vi "Sonicator Settings Dialog.vi"(8 "error in (no error)":errorcluster, 11 "Scale Module Config In":T1={"GUID"="", "Drop Coords"={"Horizontal"=0, "Vertical"=0}, "Process Name"="", "Queue Name"="", "Settings"={"Cycle Period"=500.0, "Mettler"={"VISA resource name"="", "Simulated?"=FALSE}, "Scale Type"=""}, "Load Count"=0}) -> (0 "error out":errorcluster, 1 "Cancelled?":bool=TRUE, 2 "UI Refresh Needed?":bool, 3 "Scale Module Config Out":T1={"GUID"="", "Drop Coords"={"Horizontal"=0, "Vertical"=0}, "Process Name"="", "Queue Name"="", "Settings"={"Cycle Period"=500.0, "Mettler"={"VISA resource name"="", "Simulated?"=FALSE}, "Scale Type"=""}, "Load Count"=0})   [LabVIEW 2018, in "Sonicator Module.lvlib"]
doc: "Dialog for selecting user specified settings."
uses:
  Sonicator Module.lvlib
  Feed Module/Controls/Sonicator Module Settings Cluster.ctl
  Mettler Toledo/Controls/Settings Cluster.ctl
  Feed Module/Controls/Sonicator Module Config Cluster.ctl
  <vilib>/Utility/miscctls.llb/LVPoint32TypeDef.ctl
  <vilib>/Utility/xml.llb/Write to XML File(string).vi
  Settings/Settings.lvlib
  Mettler Toledo/Mettler Toledo.lvlib
panel:
  in  "Module Name":string
  in  "Scale Configurations":T3={"Cycle Period"=500.0, "Mettler"={"VISA resource name"="", "Simulated?"=FALSE}, "Scale Type"="Default"}
  in  "Cancel Button":bool
  in  "OK Button":bool
  # "Non visible portion of dialog (needed for connector pane)."
  # "Scale Settings"
  # "Scale Settings"
  # "Scale Settings"
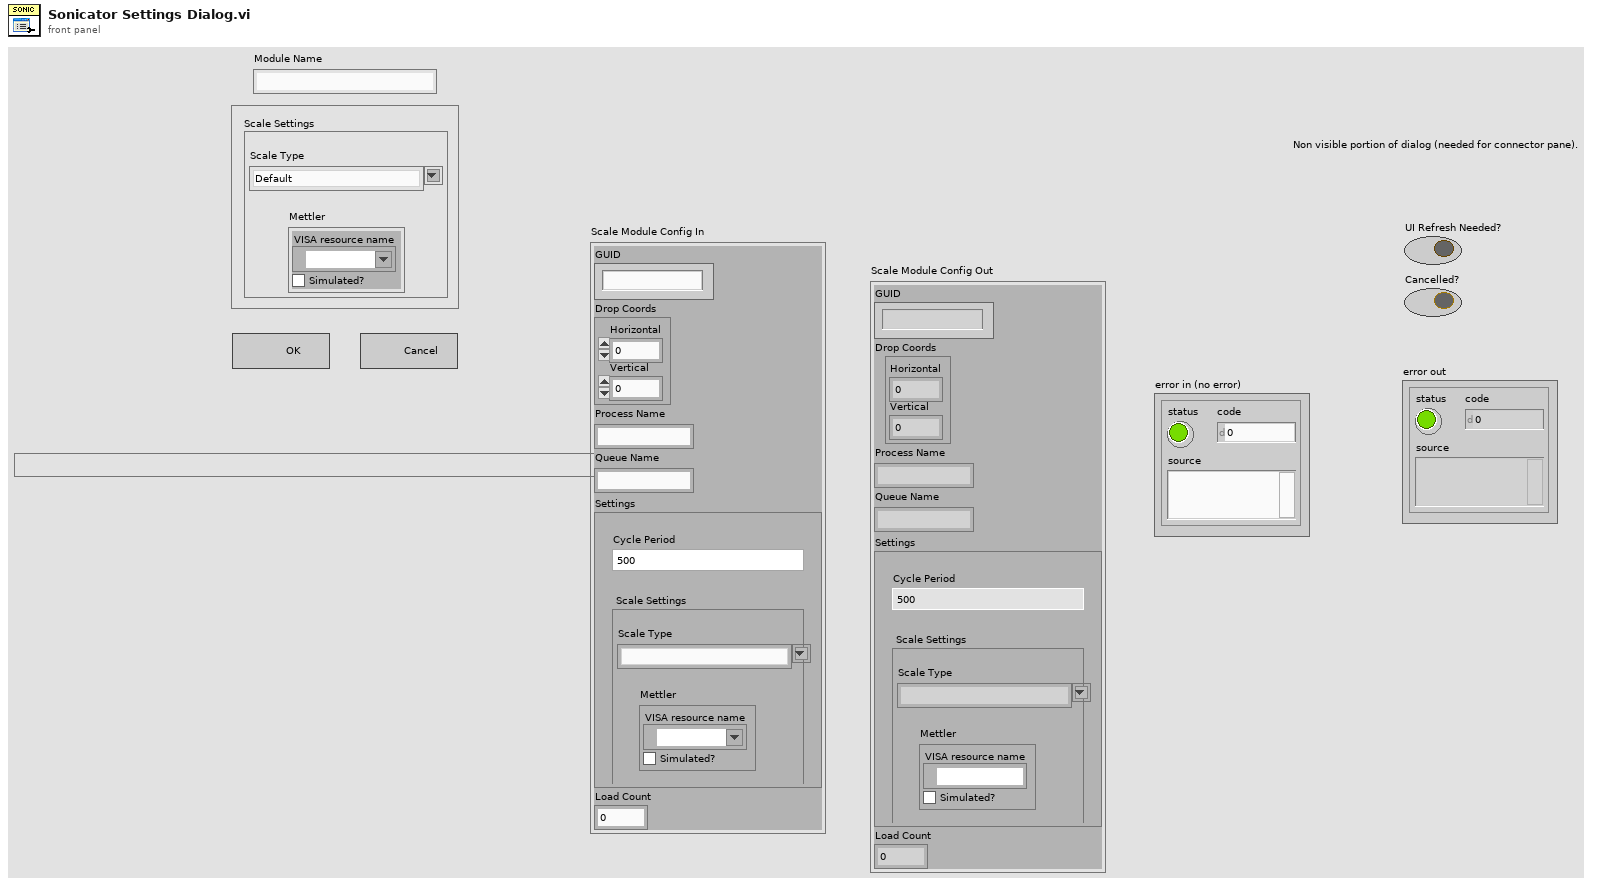
[diagram p1: front panel]
types:
  T1 = typedef "Sonicator Module.lvlib/Sonicator Module Config Cluster.ctl" = cluster{"GUID":string, "Drop Coords":T2, "Process Name":string, "Queue Name":string, "Settings":T3, "Load Count":i32}
  T2 = typedef "LVPoint32TypeDef.ctl" = cluster{"Horizontal":i32, "Vertical":i32}
  T3 = typedef "Sonicator Module.lvlib/Sonicator Module Settings Cluster.ctl" = cluster{"Cycle Period":dbl, "Mettler":T4, "Scale Type":string}
  T4 = typedef "Mettler Toledo.lvlib/Settings Cluster.ctl" = cluster{"VISA resource name":refnum<visa-resource-name>, "Simulated?":bool}
  T5 = enum8{"Enabled", "Disabled", "Disabled and Grayed Out"}
  T6 = cluster{"Cycle Period":dbl, "Mettler":T4, "Scale Type":string}
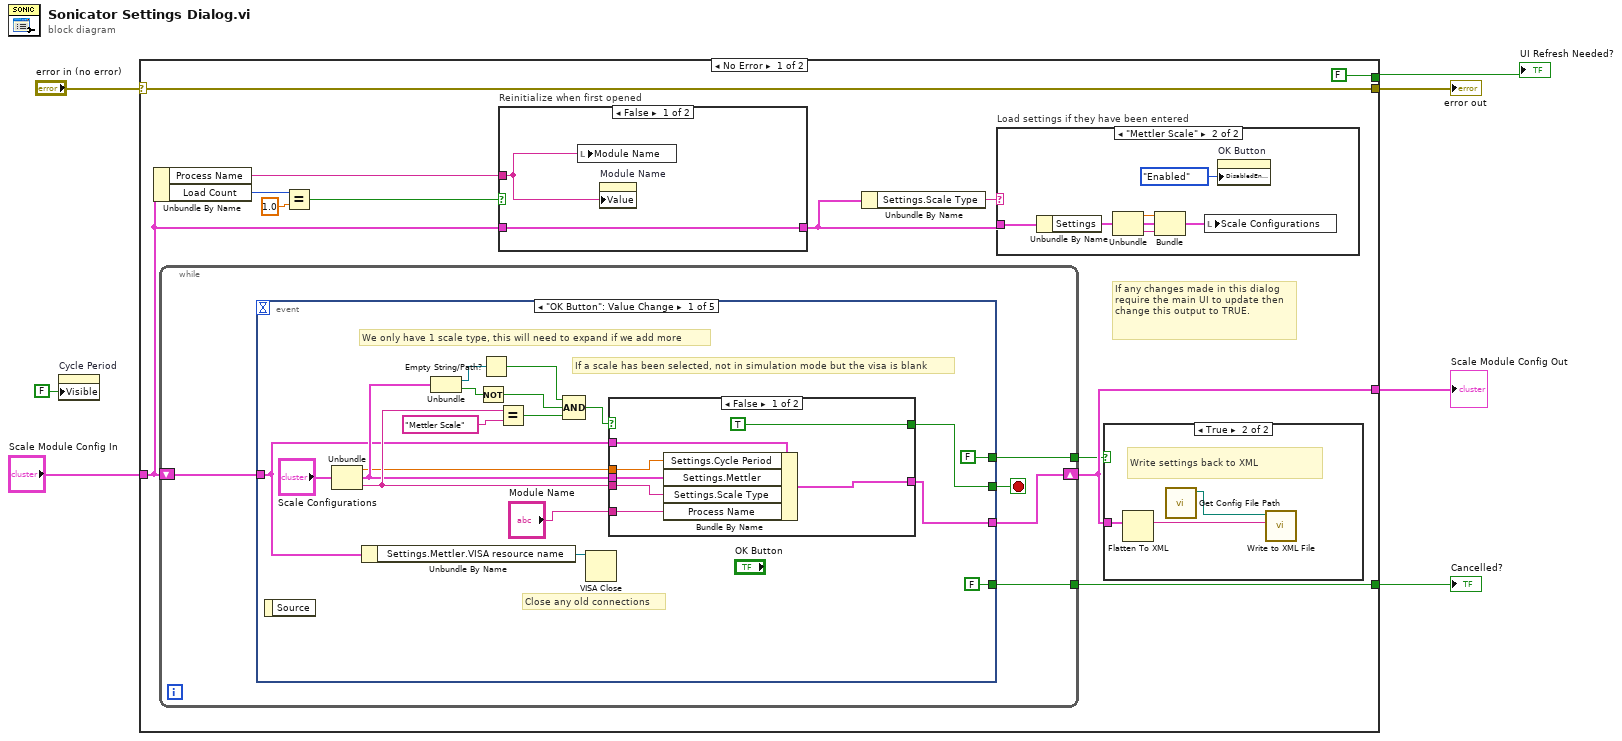
[diagram p0: block diagram]
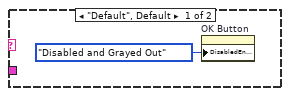
[diagram p2: hidden frame]
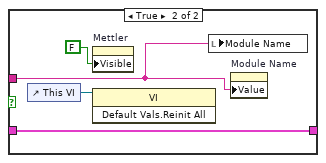
[diagram p3: hidden frame]
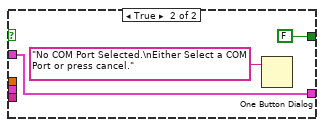
[diagram p4: hidden frame]
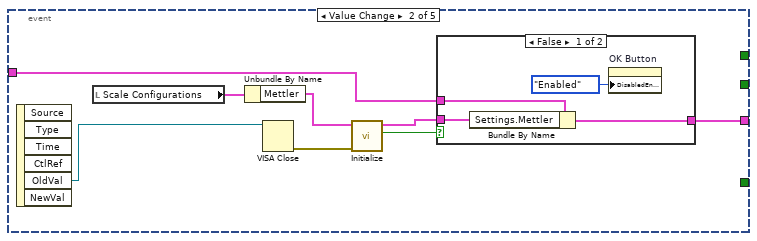
[diagram p5: hidden frame]
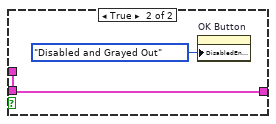
[diagram p6: hidden frame]
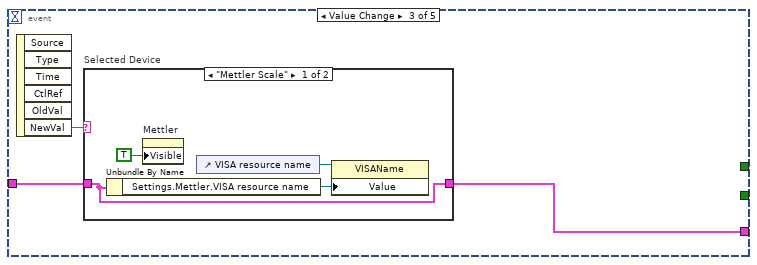
[diagram p7: hidden frame]
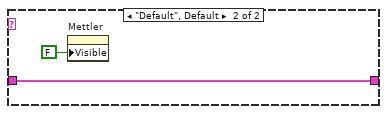
[diagram p8: hidden frame]
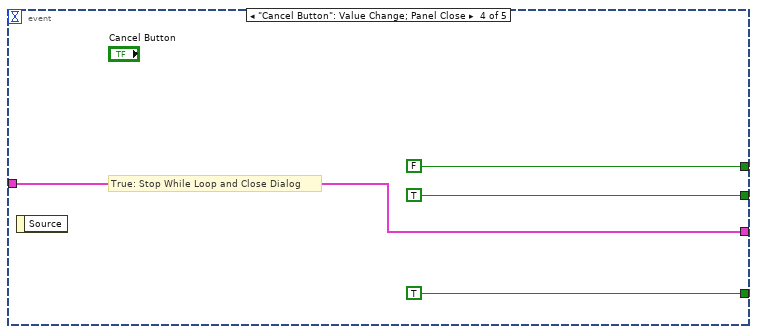
[diagram p9: hidden frame]
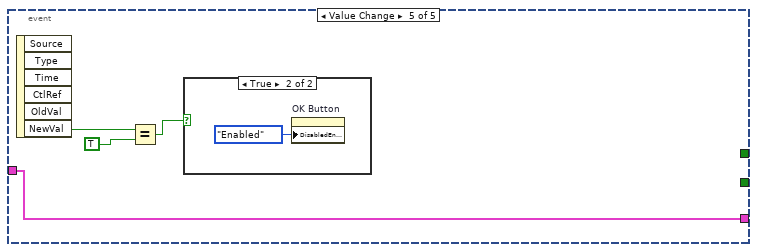
[diagram p10: hidden frame]
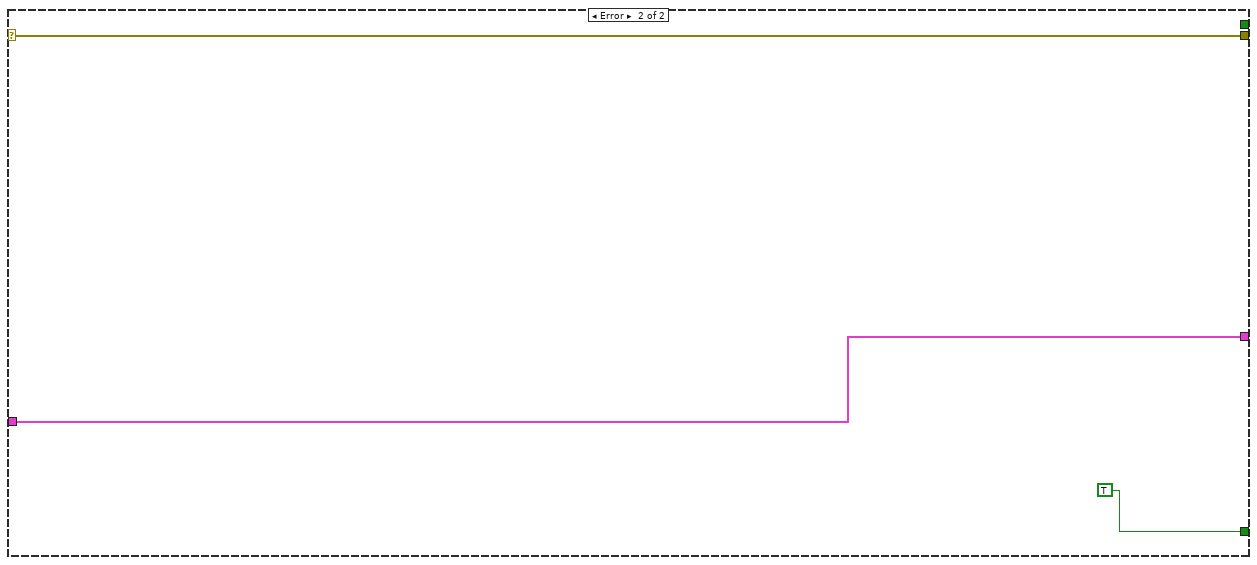
[diagram p13: hidden frame]
diagram:
  n1 = property on="Cycle Period" class="DigNum (strict)"("Visible"=FALSE) -> ()  [unwired: 2 in, 2 out]
  n2 = case shown="No Error" "error in (no error)" {
    selector: "error in (no error)" -> [w19 w104]
    tunnel: [w19 w104] -> w7
    tunnel: "Scale Module Config In" -> [w9 w103]
    tunnel: [w17 w103] -> w2
    tunnel: [FALSE ("UI Refresh Needed?") _] -> w6
    tunnel: [w13 TRUE ("UI Refresh Needed?")] -> w5
    frame No Error {
      # "If any changes made in this dialog require the main UI to update then change this output to TRUE."
      n3 = Unbundle By Name(w9) -> ("Process Name"=w8:string, "Load Count"=w16:i32)
      n4 = while {
        tunnel: [w38] -> w14
        tunnel: [w35] -> w13
        shift-right: [w37] -> w17
        shift-left: w9 -> [w34]
        stop <- w36 stop-if-true
        n5 = event shown="[0] \"OK Button\": Value Change" {
          selector: _ -> [_ _ _ _ _]
          dyn-events: _ -> [_ _ _ _ _]
          timeout: _ -> [_ _ _ _ _]
          tunnel: [w54 w72 w82 w93 w97] -> w37
          tunnel: w34 -> [w45 w73 w81 w93 w97]
          tunnel: [FALSE ("UI Refresh Needed?") _ _ FALSE ("UI Refresh Needed?") _] -> w38
          tunnel: [w55 _ _ TRUE _] -> w36
          tunnel: [FALSE ("UI Refresh Needed?") _ _ TRUE ("UI Refresh Needed?") _] -> w35
          event "OK Button": Value Change {
            # "Close any old connections"
            # "If a scale has been selected, not in simulation mode but the visa is blank"
            # "We only have 1 scale type, this will need to expand if we add more"
            n6 = event-data() -> ()  [unwired: 1 in, 1 out]
            n7 = Unbundle("Scale Configurations") -> ("Cycle Period"=w48:dbl, "Mettler"=w49:T4, "Scale Type"=w51:string)
            n8 = Unbundle By Name(w45) -> ("Settings.Mettler.VISA resource name"=w44:refnum<visa-resource-name>)
            n9 = Unbundle(w49) -> ("VISA resource name"=w52:refnum<visa-resource-name>, "Simulated?"=w47:bool)
            n10 = Not(x=w47) -> (.not. x?=w41:bool)
            n11 = Empty String/Path?(string/path=w52) -> (empty?=w42:bool)
            n12 = Equal?(x=w51, y="Mettler Scale") -> (x = y?=w40:bool)
            n13 = Compound Arithmetic op=AND(w42, w41, w40) -> (w39:bool)
            n14 = VISA Close(VISA resource name=w44) -> ()  [unwired: 1 in, 1 out]
            n15 = case shown="False" w39 {
              tunnel: [TRUE FALSE] -> w55
              tunnel: [w62 w65] -> w54
              tunnel: w45 -> [w61 w65]
              tunnel: w51 -> [w60 _]
              tunnel: w49 -> [w59 _]
              tunnel: w48 -> [w58 _]
              tunnel: "Module Name" -> [w57 _]
              frame False {
                n16 = Bundle By Name(cluster=w61, "Settings.Cycle Period"=w58, "Settings.Mettler"=w59, "Settings.Scale Type"=w60, "Process Name"=w57) -> (w62:T1)
              }
              frame True {
                n17 = One Button Dialog(message="No COM Port Selected.\nEither Select a COM Port or press cancel.") -> ()  [unwired: 1 in, 1 out]
              }
            }
          }
          event Value Change {
            n18 = event-data() -> ("OldVal"=w68:refnum<visa-resource-name>)  [unwired: 1 in, 5 out]
            n19 = local read "Scale Configurations"() -> (w74:T3)
            n20 = Unbundle By Name(w74) -> ("Mettler"=w71:T4)
            n21 = VISA Close(VISA resource name=w68) -> (error out=w69:errorcluster)  [unwired: 1 in]
            n22 = call "Initialize.vi"("error in (no error)"=w69, "Mettler Settings in"=w71) -> ("No Scale Connected"=w67:bool, "Mettler Settings out"=w70:T4)  [unwired: 7 in, 1 out]
            n23 = case shown="False" w67 {
              tunnel: w73 -> [w78 w80]
              tunnel: [w77 w80] -> w72
              tunnel: w70 -> [w76 _]
              frame False {
                n24 = Bundle By Name(cluster=w78, "Settings.Mettler"=w76) -> (w77:T1)
                n25 = property on="OK Button" class="Bool"("DisabledEnum"=T5."Enabled" ("Disabled")) -> ()  [unwired: 2 in, 2 out]
              }
              frame True {
                n26 = property on="OK Button" class="Bool"("DisabledEnum"=T5."Disabled and Grayed Out" ("Disabled")) -> ()  [unwired: 2 in, 2 out]
              }
            }
          }
          event Value Change {
            n27 = event-data() -> ("NewVal"=w83:string)  [unwired: 1 in, 5 out]
            n28 = case "Selected Device" shown="\"Mettler Scale\"" w83 {
              tunnel: [w84 w89] -> w82
              tunnel: w81 -> [w84 w89]
              frame "Mettler Scale" {
                n29 = Unbundle By Name(w84) -> ("Settings.Mettler.VISA resource name"=w87:refnum<visa-resource-name>)
                n30 = property on="Mettler" class="Clust (strict)"("Visible"=TRUE) -> ()  [unwired: 2 in, 2 out]
                n31 = control-ref of="VISA resource name"() -> (w85:refnum<vi>)
                n32 = property on="Property Node" class="VISAName"(reference=w85, "Value"=w87) -> ()  [unwired: 1 in, 2 out]
              }
              frame "Default", Default {
                n33 = property on="Mettler" class="Clust (strict)"("Visible"=FALSE) -> ()  [unwired: 2 in, 2 out]
              }
            }
          }
          event "Cancel Button": Value Change; Panel Close {
            # "True: Stop While Loop and Close Dialog"
            n34 = event-data() -> ()  [unwired: 1 in, 1 out]
          }
          event Value Change {
            n35 = event-data() -> ("NewVal"=w95:bool)  [unwired: 1 in, 5 out]
            n36 = Equal?(x=w95, y=TRUE) -> (x = y?=w94:bool)
            n37 = case shown="True" w94 {
              frame False {
              }
              frame True {
                n38 = property on="OK Button" class="Bool"("DisabledEnum"=T5."Enabled" ("Disabled")) -> ()  [unwired: 2 in, 2 out]
              }
            }
          }
        }
      }
      n39 = Equal?(x=w16, y=1.0) -> (x = y?=w12:bool)
      n40 = case "Reinitialize when first opened" shown="False" w12 {
        tunnel: w9 -> [w29 w32]
        tunnel: [w29 w32] -> w10
        tunnel: w8 -> [w28 w30]
        frame False {
          n41 = local write "Module Name"(w28) -> ()
          n42 = property on="Module Name" class="Str"("Value"=w28) -> ()  [unwired: 2 in, 2 out]
        }
        frame True {
          n43 = control-ref of="This VI"() -> (w33:refnum<vi>)
          n44 = property on="Mettler" class="Clust (strict)"("Visible"=FALSE) -> ()  [unwired: 2 in, 2 out]
          n45 = invoke class="VI" method="Default Vals.Reinit All"(reference=w33) -> ()  [unwired: 2 in, 3 out]
          n46 = local write "Module Name"(w30) -> ()
          n47 = property on="Module Name" class="Str"("Value"=w30) -> ()  [unwired: 2 in, 2 out]
        }
      }
      n48 = Unbundle By Name(w10) -> ("Settings.Scale Type"=w11:string)
      n49 = case "Load settings if they have been entered" shown="\"Mettler Scale\"" w11 {
        tunnel: w10 -> [_ w22]
        frame "Default", Default {
          n50 = property on="OK Button" class="Bool"("DisabledEnum"=T5."Disabled and Grayed Out" ("Disabled")) -> ()  [unwired: 2 in, 2 out]
        }
        frame "Mettler Scale" {
          n51 = Unbundle By Name(w22) -> ("Settings"=w24:T3)
          n52 = Unbundle(w24) -> ("Cycle Period"=w26:dbl, "Mettler"=w27:T4, "Scale Type"=w23:string)
          n53 = Bundle("Cycle Period"=w26, "Mettler"=w27, "Scale Type"=w23) -> (w25:T6)  [unwired: 1 in]
          n54 = local write "Scale Configurations"(w25) -> ()
          n55 = property on="OK Button" class="Bool"("DisabledEnum"=T5."Enabled" ("Disabled")) -> ()  [unwired: 2 in, 2 out]
        }
      }
      n56 = case shown="True" w14 {
        tunnel: w17 -> [_ w100]
        frame False {
        }
        frame True {
          # "Write settings back to XML"
          n57 = Flatten To XML(anything=w100) -> (xml string=w99:string)
          n58 = call "Get Config File Path.vi"() -> ("XML File Path"=w101:path)  [unwired: 10 in, 1 out]
          n59 = call-poly <vilib>:"Write to XML File.vi"("XML Input"=w99, "XML File Path"=w101) -> ()  [unwired: 7 in, 3 out]
        }
      }
    }
    frame Error {
    }
  }
  "UI Refresh Needed?" <- w6
  "error out" <- w7
  "Cancelled?" <- w5
  "Scale Module Config Out" <- w2
